vi "custompm.vi"() -> ()   [LabVIEW 2009]
uses:
  <vilib>/Utility/file.llb/Write To Spreadsheet File (DBL).vi
  <vilib>/Analysis/NI_AALBase.lvlib
panel:
  in  "Power Scan File Save Path":path
  in  "Save Scan":bool
  out "XY Graph":cluster{dbl[], dbl[]}(graph)
  out "Wave Cal":dbl
  in  "BWIn":u16(ring) caption="Bandwidth" items=["HIGH", "LOW"]
  in  "Averaging Rate":i32=300 min=1 max=10000 step=1
  in  "Beam\nDiameter (mm)":dbl=1.0 min=1.0 max=9.0 step=0.5
  out "RANG_Val":dbl
  out "RANG_lbl":string
  out "Rng":string
  out "AUTO?":bool
  in  "AUTO":bool
  in  "Range":i16=1 min=1 max=4 step=1
  in  "Zero?":bool
  out "ZeroValue":dbl
  out "Error log":string
  out "Readout string":string
  out "Readout value":dbl format="%^#_9e"
  out "New":bool
  in  "Close Power Meter":bool
  out "PM Visa":refnum<visa-resource-name>
  out "PM Error":errorcluster
  out "Sensor SN":string
  out "Sensor Name":string
  out "Power Meter Active?":bool
  out "IDN String":string
  in  "Use PowerMeter":bool
  out "Turning Turret":bool
  in  "Exit":bool
  in  "Abort\n Scan":bool
  out "Scanning":bool
  out "error out":errorcluster
  out "Status":string
  out "Emulating":bool
  out "Initialized":bool
  in  "Force\nInitialization":bool
  in  "Initialize":bool
  out "Current UniqueID":string
  in  "Mono ID":string(combo)
  in  "Switch \nTurret":bool
  out "Wavelength (nm)":dbl
  out "Grating Index":i32
  in  "Select Grating Blaze":string(combo)
  out "Current Blaze":string caption="Grating Blaze"
  out "Grating Density":dbl
  in  "Step Time (sec)":dbl=1.0 min=0.01 max=10.0 step=0.01
  in  "Wavelength\n   Step Size":dbl=1.0 min=0.1 max=100.0
  in  "Ending\nWavelength":dbl=500.0 min=451.0 max=2501.0
  in  "Starting\nWavelength":dbl=400.0 min=400.0 max=2500.0
  in  "Target\nWavelength":dbl=400.0 min=400.0 max=3000.0
  in  "Increment":dbl=10.0 min=0.1 max=50.0
  out "Incrementing Down":bool
  out "Incrementing Up":bool
  out "Changing Wavelength":bool
  in  "Scan":bool
  in  "Increment Down":bool
  in  "Increment Up":bool
  in  "Change Wavelength":bool
  out "Drive Control Engaged":bool
  in  "Change \nGrating":bool
  in  "Enable\nDrive":bool
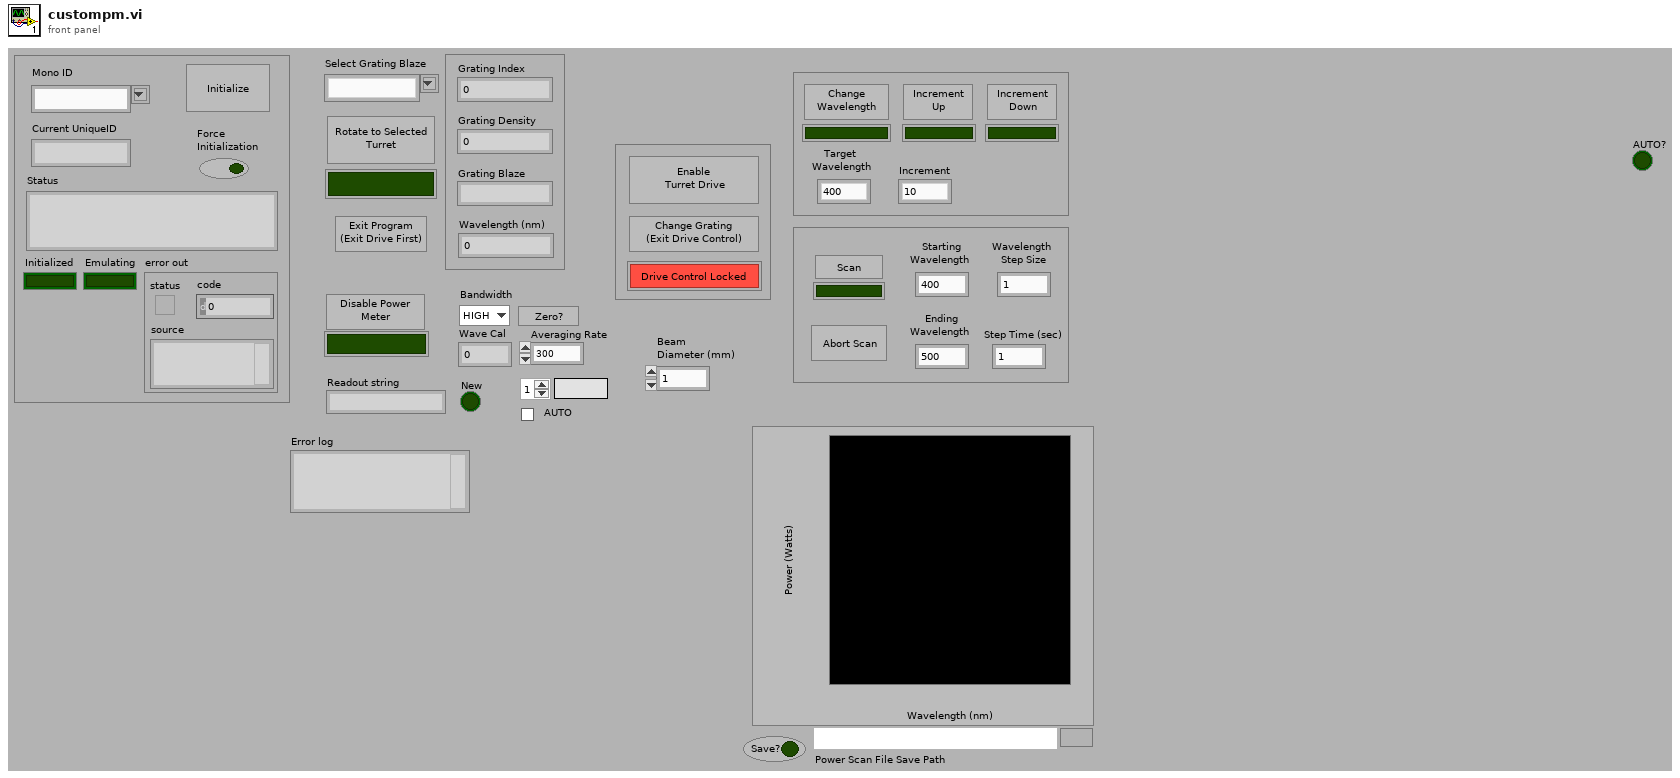
[diagram p1: front panel]
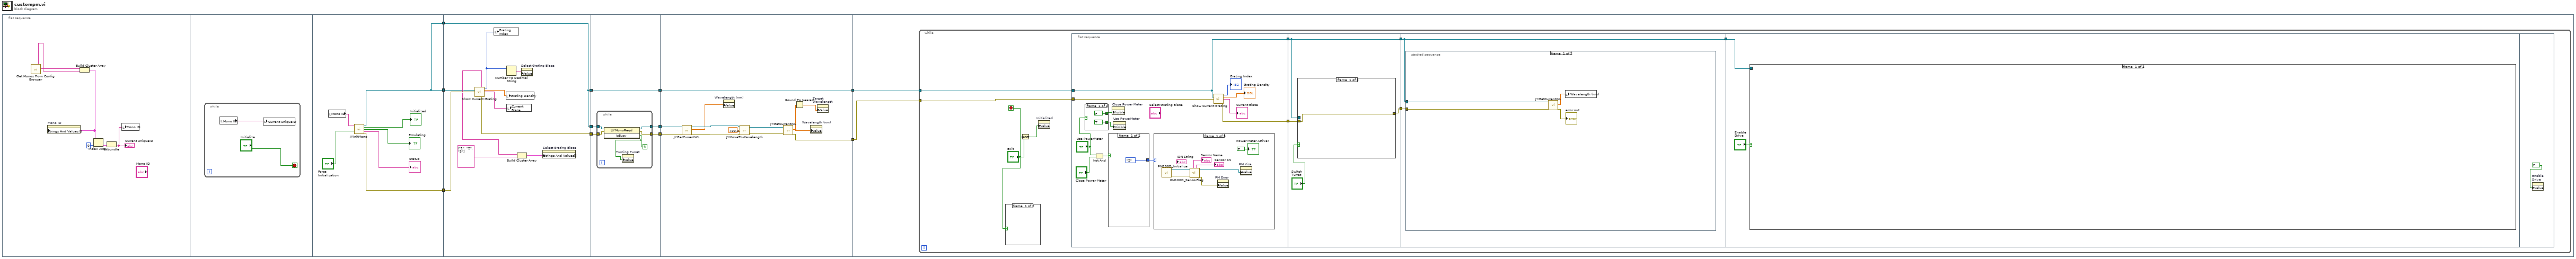
[diagram p0: block diagram]
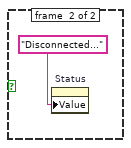
[diagram p2: hidden frame]
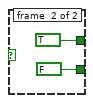
[diagram p3: hidden frame]
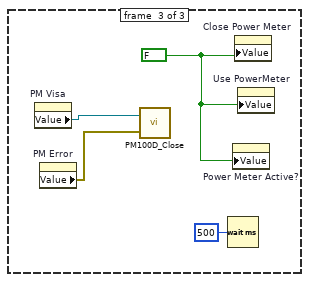
[diagram p5: hidden frame]
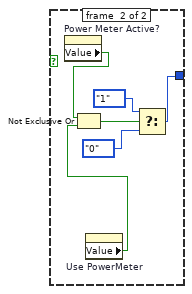
[diagram p6: hidden frame]
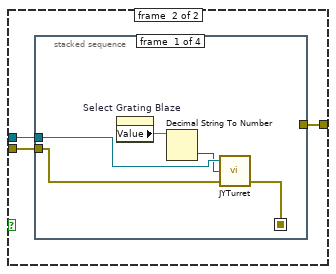
[diagram p7: hidden frame]
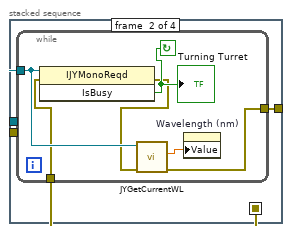
[diagram p8: hidden frame]
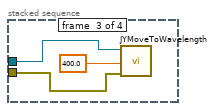
[diagram p9: hidden frame]
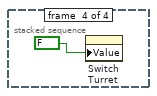
[diagram p10: hidden frame]
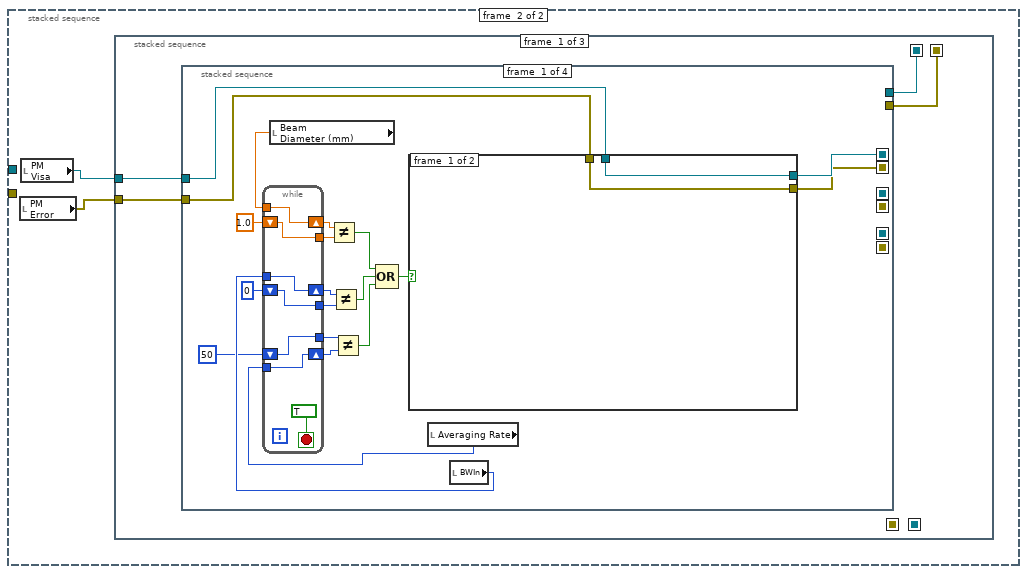
[diagram p11: hidden frame]
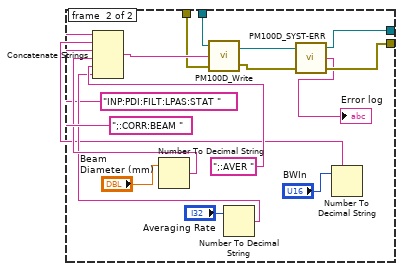
[diagram p12: hidden frame]
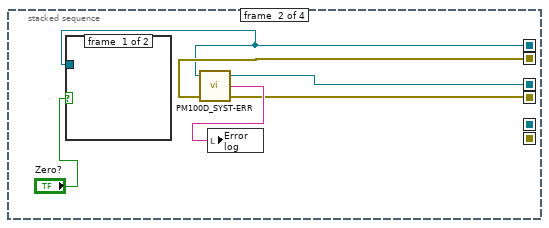
[diagram p13: hidden frame]
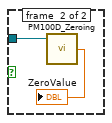
[diagram p14: hidden frame]
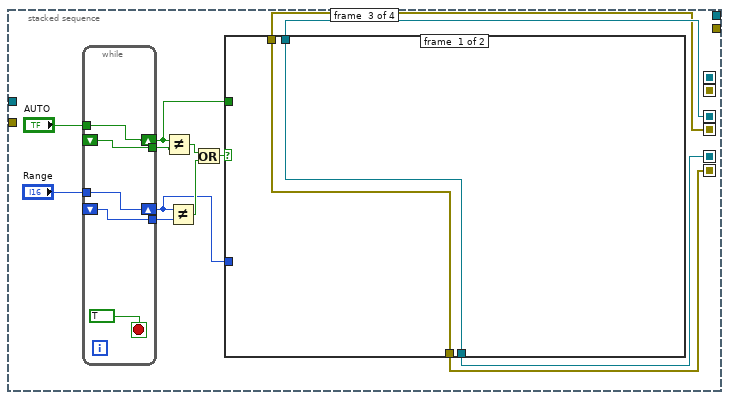
[diagram p15: hidden frame]
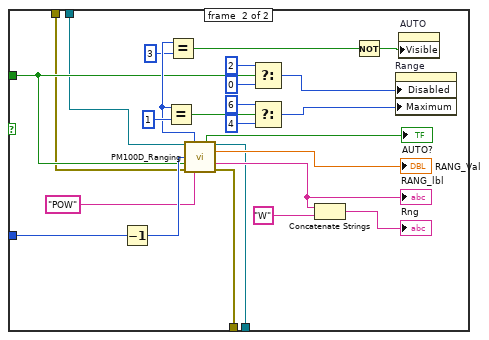
[diagram p16: hidden frame]
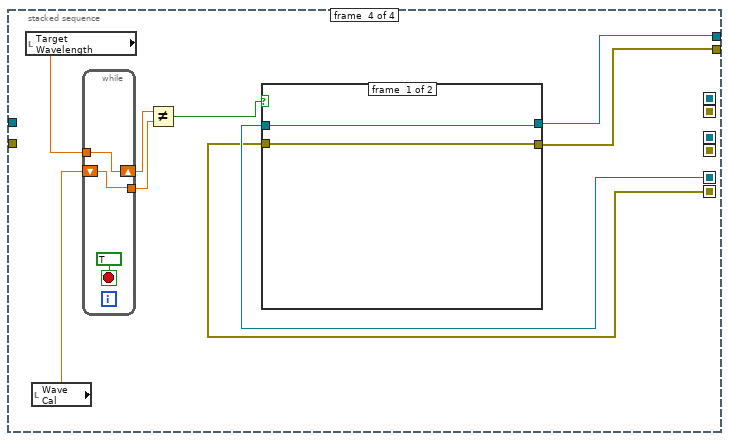
[diagram p17: hidden frame]
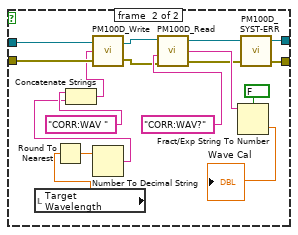
[diagram p18: hidden frame]
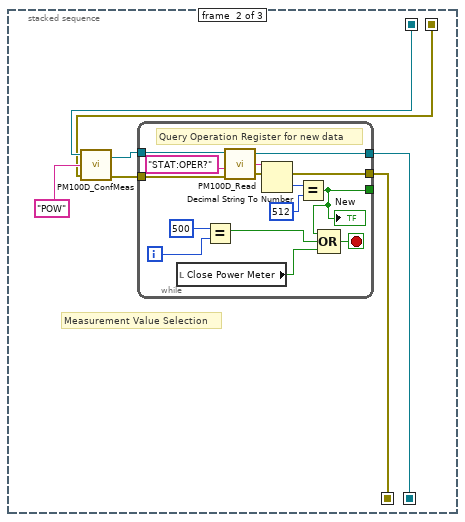
[diagram p19: hidden frame]
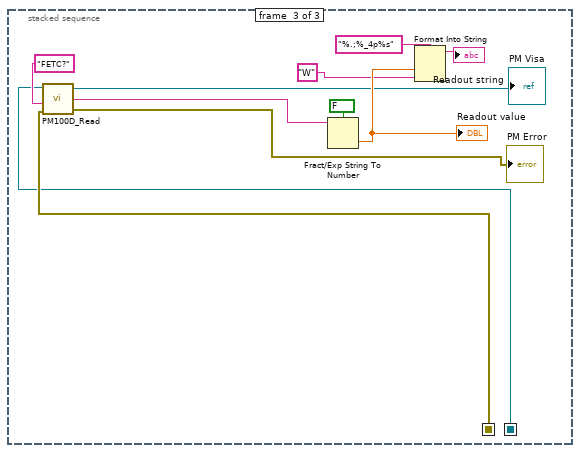
[diagram p20: hidden frame]
diagram:
  n1 = flat-sequence {
    tunnel: [w21] -> w11
    tunnel: [w20] -> w10
    tunnel: [w20] -> w7
    tunnel: w11 -> [w37]
    tunnel: w10 -> [w28]
    tunnel: [w35] -> w4
    tunnel: [w27] -> w6
    tunnel: w7 -> [w27]
    tunnel: [w27] -> w3
    tunnel: w6 -> [w41]
    tunnel: [w39] -> w5
    tunnel: w4 -> [w40]
    tunnel: w3 -> [w42]
    tunnel: [w42] -> w2
    tunnel: [w38] -> w1
    tunnel: w5 -> [w59]
    tunnel: [w57] -> w9
    tunnel: [w56] -> w8
    tunnel: w2 -> [w57]
    tunnel: w1 -> [w58]
    tunnel: w9 -> [w60]
    tunnel: w8 -> [w61]
    frame #0 {
      n2 = call "Get Monos From Config Browser.vi"() -> ("UniqueIDs"=w16:string[], "Mono ID"=w17:string[])  [unwired: 3 in, 1 out]
      n3 = Build Cluster Array(w17, w16) -> (w14:cluster{"String":string, "String":string}[])
      n4 = property on="Mono ID" class="CmbBox"("Strings And Values []"=w14) -> ()  [unwired: 2 in, 2 out]
      n5 = Index Array(array=w14, index=0) -> (element=w15:cluster{"String":string, "String":string})
      n6 = Unbundle(w15) -> ("String"=w12:string)  [unwired: 1 out]
      "Current UniqueID" <- w12
      n7 = local write "Mono ID"(w12) -> ()
    }
    frame #1 {
      n8 = while {
        stop <- "Initialize" stop-if-true
        n9 = local read "Mono ID"() -> (w19:string)
        n10 = local write "Current UniqueID"(w19) -> ()
      }
    }
    frame #2 {
      n11 = local read "Mono ID"() -> (w25:string)
      n12 = call "JYInitMono.vi"("Unique ID"=w25, "Force Init"="Force\nInitialization") -> ("Mono RefNum out"=w20:refnum<k7>, "Initialized"=→"Initialized":bool, "Emulating"=→"Emulating":bool, "Status"=→"Status":string, "error out"=w21:errorcluster)  [unwired: 9 in]
    }
    frame #3 {
      n13 = call "Show Current Grating.vi"("Refnum in"=w28, "error in (no error)"=w37) -> ("Blazes"=w32:string[], "Grating Index"=w31:i32, "Current Grating"=w30:dbl, "Current Blaze"=w29:string, "error out"=w35:errorcluster)  [unwired: 5 in, 4 out]
      n14 = local write "Grating Index"(w31) -> ()
      n15 = local write "Grating Density"(w30) -> ()
      n16 = Number To Decimal String(number=w31) -> (decimal integer string=w34:string)  [unwired: 1 in]
      n17 = local write "Current Blaze"(w29) -> ()
      n18 = Build Cluster Array(w32, string[] ["1", "2", "3"]) -> (w33:cluster{"String":string, string}[])
      n19 = property on="Select Grating Blaze" class="CmbBox"("Value"=w34) -> ()  [unwired: 2 in, 2 out]
      n20 = property on="Select Grating Blaze" class="CmbBox"("Strings And Values[]"=w33) -> ()  [unwired: 2 in, 2 out]
    }
    frame #4 {
      n21 = while {
        tunnel: w41 -> [w47]
        tunnel: w40 -> [w46]
        tunnel: [w45] -> w39
        tunnel: [w44] -> w38
        stop <- w43 continue-if-true
        n22 = invoke class="IJYMonoReqd" method="IsBusy"(reference=w47, error in=w46) -> (reference out=w45:refnum<k7>, error out=w44:errorcluster, "IsBusy"=w43:bool)  [unwired: 1 in]
        n23 = property on="Turning Turret" class="Bool (strict)"("Value"=w43) -> ()  [unwired: 2 in, 2 out]
      }
    }
    frame #5 {
      n24 = call "JYGetCurrentWL.vi"("error in (no error)"=w58, "JYMONOLib.IJYMonoReqd"=w59) -> ("error out"=w53:errorcluster, "Current WL"=w49:dbl, "Mono Refnum Out"=w54:refnum<k7>)  [unwired: 6 in, 1 out]
      n25 = property on="Wavelength (nm)" class="DigNum (strict)"("Value"=w49) -> ()  [unwired: 2 in, 2 out]
      n26 = call "JYMoveToWavelength.vi"("error in (no error)"=w53, "Target WL"=400.0, "RefNum In"=w54) -> ("error out"=w51:errorcluster, "Refnum Out"=w52:refnum<k7>)  [unwired: 1 in, 1 out]
      n27 = call "JYGetCurrentWL.vi"("error in (no error)"=w51, "JYMONOLib.IJYMonoReqd"=w52) -> ("error out"=w56:errorcluster, "Current WL"=w50:dbl)  [unwired: 6 in, 2 out]
      n28 = Round To Nearest(number=w50) -> (nearest integer value=w48:dbl)
      n29 = property on="Wavelength (nm)" class="DigNum (strict)"("Value"=w50) -> ()  [unwired: 2 in, 2 out]
      n30 = property on="Target\nWavelength" class="DigNum (strict)"("Value"=w48) -> ()  [unwired: 2 in, 2 out]
    }
    frame #6 {
      n31 = while {
        tunnel: w60 -> [w70]
        tunnel: w61 -> [w69]
        stop <- "Exit" stop-if-true
        n32 = case shown="True" "Exit" {
          frame #0 {
          }
          frame #1 {
            n33 = property on="Status" class="Str"("Value"="Disconnected...") -> ()  [unwired: 2 in, 2 out]
          }
        }
        n34 = Not(x="Exit") -> (.not. x?=w62:bool)
        n35 = property on="Initialized" class="Bool (strict)"("Value"=w62) -> ()  [unwired: 2 in, 2 out]
        n36 = flat-sequence {
          tunnel: w70 -> [w78]
          tunnel: w69 -> [w80]
          tunnel: [w79] -> w68
          tunnel: [w78] -> w66
          tunnel: w68 -> [w109]
          tunnel: [w107] -> w67
          tunnel: w66 -> [w108]
          tunnel: [w108] -> w65
          tunnel: w67 -> [w133]
          tunnel: w65 -> [w132]
          tunnel: [w132] -> w64
          tunnel: w64 -> [w307]
          frame #0 {
            n37 = case shown="True" "Use PowerMeter" {
              tunnel: [FALSE TRUE] -> w72
              tunnel: [TRUE FALSE] -> w73
              frame #0 {
              }
              frame #1 {
              }
            }
            n38 = Not And(1:"Close Power Meter", 2:"Use PowerMeter") -> (0:w76:bool)
            n39 = case shown="True" w76 {
              tunnel: [enum16{"0", "1", "2"}."2" w102] -> w75
              frame #0 {
              }
              frame #1 {
                n40 = property on="Power Meter Active?" class="Bool (strict)"() -> ("Value"=w100:bool)  [unwired: 2 in, 2 out]
                n41 = property on="Use PowerMeter" class="Bool (strict)"() -> ("Value"=w101:bool)  [unwired: 2 in, 2 out]
                n42 = Not Exclusive Or(1:w101, 2:w100) -> (0:w103:bool)
                n43 = Select(t=enum16{"0", "1", "2"}."1", s=w103, f=enum16{"0", "1", "2"}."0") -> (s? t:f=w102:enum16{"0", "1", "2"})
              }
            }
            n44 = property on="Close Power Meter" class="Bool (strict)"("Visible"=w72) -> ()  [unwired: 2 in, 2 out]
            n45 = property on="Use PowerMeter" class="Bool (strict)"("Visible"=w73) -> ()  [unwired: 2 in, 2 out]
            n46 = case shown="\"2\"" w75 {
              frame #0 {
                n47 = call "PM100D_Initialize.vi"() -> ("error out"=w92:errorcluster, "VISA out"=w93:refnum<visa-resource-name>)  [unwired: 2 in, 2 out]
                n48 = call "PM100D_SensorFlag.vi"("error in (no error)"=w92, "VISA in"=w93) -> ("error out"=w89:errorcluster, "VISA out"=w88:refnum<visa-resource-name>, "sn"=→"Sensor SN":string, "name"=→"Sensor Name":string)  [unwired: 2 in, 4 out]
                n49 = property on="PM Error" class="Clust (strict)"("Value"=w89) -> ()  [unwired: 2 in, 2 out]
                n50 = property on="PM Visa" class="VISAName"("Value"=w88) -> ()  [unwired: 2 in, 2 out]
                "Power Meter Active?" <- TRUE ("Power Meter Active?")
              }
              frame #1 {
              }
              frame #2 {
                w96 = FALSE
                n51 = property on="PM Visa" class="VISAName"() -> ("Value"=w98:refnum<visa-resource-name>)  [unwired: 2 in, 2 out]
                n52 = property on="PM Error" class="Clust (strict)"() -> ("Value"=w97:errorcluster)  [unwired: 2 in, 2 out]
                n53 = call "PM100D_Close.vi"("error in (no error)"=w97, "VISA resource name"=w98) -> ()  [unwired: 2 in]
                n54 = Wait (ms)(milliseconds to wait=u32 500) -> ()  [unwired: 1 out]
                n55 = property on="Power Meter Active?" class="Bool (strict)"("Value"=w96) -> ()  [unwired: 2 in, 2 out]
                n56 = property on="Close Power Meter" class="Bool (strict)"("Value"=w96) -> ()  [unwired: 2 in, 2 out]
                n57 = property on="Use PowerMeter" class="Bool (strict)"("Value"=w96) -> ()  [unwired: 2 in, 2 out]
              }
            }
            n58 = call "Show Current Grating.vi"("Refnum in"=w78, "error in (no error)"=w80) -> ("Grating Index"=→"Grating Index":i32, "Current Grating"=→"Grating Density":dbl, "Current Blaze"=→"Current Blaze":string, "error out"=w79:errorcluster)  [unwired: 5 in, 5 out]
          }
          frame #1 {
            n59 = case shown="True" "Switch \nTurret" {
              tunnel: w109 -> [w110 w113]
              tunnel: w108 -> [_ w112]
              tunnel: [w110 w111] -> w107
              frame #0 {
              }
              frame #1 {
                n60 = stacked-sequence {
                  seq-local: [w116 _ _ _] -> [_ w120 _ _]
                  tunnel: w113 -> [w118 _ w129 _]
                  tunnel: w112 -> [w117 w121 w128 _]
                  tunnel: [_ w119 _ _] -> w111
                  frame #0 {
                    n61 = property on="Select Grating Blaze" class="CmbBox"() -> ("Value"=w115:string)  [unwired: 2 in, 2 out]
                    n62 = Decimal String To Number(string=w115) -> (number=w114:i32)  [unwired: 2 in, 1 out]
                    n63 = call "JYTurret.vi"("error in (no error)"=w118, "Grating Index"=w114, "RefNum In"=w117) -> ("error out"=w116:errorcluster)  [unwired: 2 out]
                  }
                  frame #1 {
                    n64 = while {
                      tunnel: w121 -> [w127]
                      tunnel: w120 -> [w126]
                      tunnel: [w123] -> w119
                      stop <- w125 continue-if-true
                      n65 = invoke class="IJYMonoReqd" method="IsBusy"(reference=w127, error in=w126) -> (error out=w124:errorcluster, "IsBusy"=w125:bool)  [unwired: 1 in, 1 out]
                      "Turning Turret" <- w125
                      n66 = call "JYGetCurrentWL.vi"("error in (no error)"=w124, "JYMONOLib.IJYMonoReqd"=w127) -> ("error out"=w123:errorcluster, "Current WL"=w122:dbl)  [unwired: 6 in, 2 out]
                      n67 = property on="Wavelength (nm)" class="DigNum (strict)"("Value"=w122) -> ()  [unwired: 2 in, 2 out]
                    }
                  }
                  frame #2 {
                    n68 = call "JYMoveToWavelength.vi"("error in (no error)"=w129, "Target WL"=400.0, "RefNum In"=w128) -> ()  [unwired: 1 in, 3 out]
                  }
                  frame #3 {
                    n69 = property on="Switch \nTurret" class="Bool (strict)"("Value"=FALSE ("Switch \nTurret")) -> ()  [unwired: 2 in, 2 out]
                  }
                }
              }
            }
          }
          frame #2 {
            n70 = stacked-sequence {
              tunnel: w133 -> [w137 _]
              tunnel: w132 -> [w136 _]
              frame #0 {
                n71 = call "JYGetCurrentWL.vi"("error in (no error)"=w137, "JYMONOLib.IJYMonoReqd"=w136) -> ("error out"=→"error out":errorcluster, "Current WL"=w134:dbl)  [unwired: 6 in, 2 out]
                n72 = local write "Wavelength (nm)"(w134) -> ()
              }
              frame #1 {
                n73 = local read "PM Error"() -> (w138:errorcluster)
                n74 = local read "PM Visa"() -> (w139:refnum<visa-resource-name>)
                n75 = stacked-sequence {
                  seq-local: [_ w278 _] -> [_ _ w299]
                  seq-local: [_ w277 _] -> [_ _ w298]
                  seq-local: [w141 _ _] -> [_ w275 _]
                  seq-local: [w140 _ _] -> [_ w274 _]
                  tunnel: w139 -> [w143 _ _]
                  tunnel: w138 -> [w142 _ _]
                  frame #0 {
                    n76 = stacked-sequence {
                      seq-local: [w163 _ _ _] -> [_ w193 _ _]
                      seq-local: [w162 _ _ _] -> [_ w194 _ _]
                      seq-local: [_ w191 _ _] -> [_ _ w201 _]
                      seq-local: [_ w190 _ _] -> [_ _ w200 _]
                      seq-local: [_ _ w199 _] -> [_ _ _ w248]
                      seq-local: [_ _ w198 _] -> [_ _ _ w247]
                      tunnel: w143 -> [w161 _ _ _]
                      tunnel: w142 -> [w160 _ _ _]
                      tunnel: [_ _ _ w246] -> w141
                      tunnel: [_ _ _ w245] -> w140
                      frame #0 {
                        n77 = local read "Beam\nDiameter (mm)"() -> (w158:dbl)
                        n78 = local read "Averaging Rate"() -> (w157:i32)
                        n79 = local read "BWIn"() -> (w156:u16)
                        n80 = while {
                          shift-right: [w188] -> w154
                          shift-left: 1.0 ("Beam\nDiameter (mm)") -> [w187]
                          shift-right: [w184] -> w152
                          shift-left: u16 0 ("BWIn") -> [w183]
                          shift-right: [w186] -> w150
                          shift-left: 50 ("Averaging Rate") -> [w185]
                          tunnel: w158 -> [w188]
                          tunnel: [w187] -> w155
                          tunnel: w157 -> [w186]
                          tunnel: [w185] -> w151
                          tunnel: w156 -> [w184]
                          tunnel: [w183] -> w153
                          stop <- TRUE stop-if-true
                        }
                        n81 = Not Equal?(x=w154, y=w155) -> (x != y?=w147:bool)
                        n82 = Not Equal?(x=w152, y=w153) -> (x != y?=w148:bool)
                        n83 = Not Equal?(x=w151, y=w150) -> (x != y?=w149:bool)
                        n84 = Compound Arithmetic op=OR(w147, w148, w149) -> (w159:bool)
                        n85 = case shown="True" w159 {
                          tunnel: [w164 w179] -> w163
                          tunnel: [w165 w178] -> w162
                          tunnel: w161 -> [w164 w167]
                          tunnel: w160 -> [w165 w166]
                          frame #0 {
                          }
                          frame #1 {
                            n86 = Number To Decimal String(number="Beam\nDiameter (mm)") -> (decimal integer string=w175:string)  [unwired: 1 in]
                            n87 = Number To Decimal String(number="Averaging Rate") -> (decimal integer string=w171:string)  [unwired: 1 in]
                            n88 = Number To Decimal String(number="BWIn") -> (decimal integer string=w168:string)  [unwired: 1 in]
                            n89 = Concatenate Strings("INP:PDI:FILT:LPAS:STAT ", w168, ";:CORR:BEAM " ("string"), w175, ";:AVER " ("string"), w171) -> (w182:string)
                            n90 = call "PM100D_Write.vi"("error in (no error)"=w166, "Command"=w182, "VISA in"=w167) -> ("error out"=w180:errorcluster, "VISA out"=w181:refnum<visa-resource-name>)
                            n91 = call "PM100D_SYST-ERR.vi"("error out 2"=w180, "VISA In"=w181) -> ("error out"=w178:errorcluster, "Error"=→"Error log":string, "VISA Out"=w179:refnum<visa-resource-name>)  [unwired: 1 in]
                          }
                        }
                      }
                      frame #1 {
                        n92 = case shown="True" "Zero?" {
                          tunnel: w193 -> [_ w197]
                          frame #0 {
                          }
                          frame #1 {
                            n93 = call "PM100D_Zeroing.vi"("VISA In"=w197) -> ("ZeroValue"=→"ZeroValue":dbl)  [unwired: 4 in]
                          }
                        }
                        n94 = call "PM100D_SYST-ERR.vi"("error out 2"=w194, "VISA In"=w193) -> ("error out"=w190:errorcluster, "Error"=w195:string, "VISA Out"=w191:refnum<visa-resource-name>)  [unwired: 1 in]
                        n95 = local write "Error log"(w195) -> ()
                      }
                      frame #2 {
                        n96 = while {
                          shift-right: [w240] -> w202
                          shift-left: _ -> [w239]
                          shift-right: [w242] -> w203
                          shift-left: _ -> [w241]
                          tunnel: "AUTO" -> [w242]
                          tunnel: [w241] -> w209
                          tunnel: "Range" -> [w240]
                          tunnel: [w239] -> w206
                          stop <- TRUE stop-if-true
                        }
                        n97 = Not Equal?(x=w203, y=w209) -> (x != y?=w208:bool)
                        n98 = Not Equal?(x=w202, y=w206) -> (x != y?=w205:bool)
                        n99 = Or(x=w208, y=w205) -> (x .or. y?=w204:bool)
                        n100 = case shown="True" w204 {
                          tunnel: w203 -> [_ w220]
                          tunnel: w202 -> [_ w219]
                          tunnel: w201 -> [w211 w217]
                          tunnel: w200 -> [w212 w215]
                          tunnel: [w211 w214] -> w199
                          tunnel: [w212 w213] -> w198
                          frame #0 {
                          }
                          frame #1 {
                            n101 = Decrement(x=w219) -> (x-1=w227:i16)
                            n102 = call "PM100D_Ranging.vi"("VISA in"=w217, "Index"=w227, "AUTO"=w220, "error in (no error)"=w215, "Unit"="POW") -> ("SensType"=w226:i32, "AUTO?"=→"AUTO?":bool, "VISA out"=w214:refnum<visa-resource-name>, "RANG_Val"=→"RANG_Val":dbl, "RANG_lbl"=w235:string, "error out"=w213:errorcluster)  [unwired: 3 in, 2 out]
                            "RANG_lbl" <- w235
                            n103 = Equal?(x=w226, y=1) -> (x = y?=w231:bool)
                            n104 = Equal?(x=w226, y=3) -> (x = y?=w221:bool)
                            n105 = Select(t=2, s=w220, f=0) -> (s? t:f=w233:i32)
                            n106 = Select(t=6, s=w231, f=4) -> (s? t:f=w232:i32)
                            n107 = Concatenate Strings(w235, "W") -> (→"Rng":string)
                            n108 = Not(x=w221) -> (.not. x?=w222:bool)
                            n109 = property on="Range" class="DigNum (strict)"("Disabled"=w233, "Maximum"=w232) -> ()  [unwired: 2 in, 2 out]
                            n110 = property on="AUTO" class="Bool (strict)"("Visible"=w222) -> ()  [unwired: 2 in, 2 out]
                          }
                        }
                      }
                      frame #3 {
                        n111 = local read "Target\nWavelength"() -> (w243:dbl)
                        n112 = local read "Wave Cal"() -> (w244:dbl)
                        n113 = while {
                          shift-right: [w272] -> w251
                          shift-left: w244 -> [w271]
                          tunnel: w243 -> [w272]
                          tunnel: [w271] -> w250
                          stop <- TRUE stop-if-true
                        }
                        n114 = Not Equal?(x=w251, y=w250) -> (x != y?=w249:bool)
                        n115 = case shown="True" w249 {
                          tunnel: w248 -> [w253 w268]
                          tunnel: w247 -> [w252 w267]
                          tunnel: [w253 w266] -> w246
                          tunnel: [w252 w265] -> w245
                          frame #0 {
                          }
                          frame #1 {
                            n116 = local read "Target\nWavelength"() -> (w254:dbl)
                            n117 = Round To Nearest(number=w254) -> (nearest integer value=w270:dbl)
                            n118 = Number To Decimal String(number=w270) -> (decimal integer string=w263:string)  [unwired: 1 in]
                            n119 = Concatenate Strings("CORR:WAV " ("string"), w263) -> (w264:string)
                            n120 = call "PM100D_Write.vi"("error in (no error)"=w267, "Command"=w264, "VISA in"=w268) -> ("error out"=w257:errorcluster, "VISA out"=w258:refnum<visa-resource-name>)
                            n121 = call "PM100D_Read.vi"("error in (no error)"=w257, "Command"="CORR:WAV?", "VISA in"=w258) -> ("error out"=w255:errorcluster, "ReadValue"=w259:string, "VISA out"=w256:refnum<visa-resource-name>)  [unwired: 1 in]
                            n122 = Fract/Exp String To Number(use system decimal point (T)=FALSE, string=w259) -> (number=→"Wave Cal":dbl)  [unwired: 2 in, 1 out]
                            n123 = call "PM100D_SYST-ERR.vi"("error out 2"=w255, "VISA In"=w256) -> ("error out"=w265:errorcluster, "VISA Out"=w266:refnum<visa-resource-name>)  [unwired: 1 in, 1 out]
                          }
                        }
                      }
                    }
                  }
                  frame #1 {
                    # "Measurement Value Selection"
                    n124 = call "PM100D_ConfMeas.vi"("error in"=w274, "Conf:"="POW", "VISA In"=w275) -> ("error out"=w279:errorcluster, "dup VISA session"=w280:refnum<visa-resource-name>)
                    n125 = while {
                      tunnel: w280 -> [w290]
                      tunnel: w279 -> [w289]
                      tunnel: [w288] -> w277
                      tunnel: [w287] -> w278
                      tunnel: [w283] -> _
                      i -> [w285]
                      stop <- w286 stop-if-true
                      # "Query Operation Register for new data"
                      n126 = local read "Close Power Meter"() -> (w282:bool)
                      n127 = Equal?(x=500, y=w285) -> (x = y?=w284:bool)
                      n128 = call "PM100D_Read.vi"("error in (no error)"=w289, "Command"="STAT:OPER?", "VISA in"=w290) -> ("error out"=w287:errorcluster, "ReadValue"=w293:string, "VISA out"=w288:refnum<visa-resource-name>)  [unwired: 1 in]
                      n129 = Decimal String To Number(string=w293) -> (number=w292:i32)  [unwired: 2 in, 1 out]
                      n130 = Equal?(x=w292, y=512) -> (x = y?=w283:bool)
                      "New" <- w283
                      n131 = Compound Arithmetic op=OR(w283, w284, w282) -> (w286:bool)
                    }
                  }
                  frame #2 {
                    n132 = call "PM100D_Read.vi"("error in (no error)"=w299, "Command"="FETC?", "VISA in"=w298) -> ("error out"=→"PM Error":errorcluster, "ReadValue"=w304:string, "VISA out"=→"PM Visa":refnum<visa-resource-name>)  [unwired: 1 in]
                    n133 = Fract/Exp String To Number(use system decimal point (T)=FALSE, string=w304) -> (number=w301:dbl)  [unwired: 2 in, 1 out]
                    "Readout value" <- w301
                    n134 = Format Into String(format string="%.;%_4p%s", w301, "W") -> (resulting string=→"Readout string":string)  [unwired: 2 in, 1 out]
                  }
                }
              }
            }
          }
          frame #3 {
            n135 = case shown="True" "Enable\nDrive" {
              selector: "Enable\nDrive" -> [_ w308]
              tunnel: w307 -> [_ w309]
              frame #0 {
              }
              frame #1 {
                n136 = while {
                  tunnel: w308 -> [w311]
                  tunnel: w309 -> [w310]
                  stop <- "Change \nGrating" stop-if-true
                  n137 = Not And(1:"Change \nGrating", 2:w311) -> (0:→"Drive Control Engaged":bool)
                  n138 = stacked-sequence {
                    seq-local: [_ "Change Wavelength" _ _ _ _] -> [_ _ w334 w353 _ _]
                    seq-local: [_ _ "Increment Up" _ _ _] -> [_ _ _ w352 _ _]
                    seq-local: [_ _ _ w347 _ _] -> [_ _ _ _ w368 _]
                    seq-local: [_ _ _ w346 _ _] -> [_ _ _ _ w367 _]
                    seq-local: [w315 _ _ _ _ _] -> [_ w320 _ _ _ _]
                    seq-local: [_ w318 _ _ _ _] -> [_ _ w330 _ _ _]
                    seq-local: [_ _ w328 _ _ _] -> [_ _ _ w345 _ _]
                    seq-local: [_ _ _ w343 _ _] -> [_ _ _ _ w363 _]
                    tunnel: w310 -> [w314 w319 w329 w344 w362 _]
                    frame #0 {
                      n139 = local read "error out"() -> (w317:errorcluster)
                      n140 = call "JYGetCurrentWL.vi"("error in (no error)"=w317, "JYMONOLib.IJYMonoReqd"=w314) -> ("error out"=w315:errorcluster, "Current WL"=→"Wavelength (nm)":dbl)  [unwired: 6 in, 2 out]
                    }
                    frame #1 {
                      n141 = case shown="True" "Change Wavelength" {
                        selector: "Change Wavelength" -> [_ w324]
                        tunnel: w320 -> [w322 w327]
                        tunnel: w319 -> [_ w326]
                        tunnel: [w322 w325] -> w318
                        frame #0 {
                        }
                        frame #1 {
                          n142 = property on="Target\nWavelength" class="DigNum (strict)"() -> ("Value"=w323:dbl)  [unwired: 2 in, 2 out]
                          n143 = call "JYMoveToWavelength.vi"("error in (no error)"=w327, "Target WL"=w323, "RefNum In"=w326) -> ("error out"=w325:errorcluster)  [unwired: 1 in, 2 out]
                          "Changing Wavelength" <- w324
                        }
                      }
                    }
                    frame #2 {
                      n144 = Not(x=w334) -> (.not. x?=w331:bool)
                      n145 = And(x="Increment Up", y=w331) -> (x .and. y?=w333:bool)
                      n146 = case shown="True" w333 {
                        selector: w333 -> [_ w339]
                        tunnel: w330 -> [w335 w342]
                        tunnel: w329 -> [_ w341]
                        tunnel: [w335 w340] -> w328
                        frame #0 {
                        }
                        frame #1 {
                          n147 = property on="Increment" class="DigNum (strict)"() -> ("Value"=w338:dbl)  [unwired: 2 in, 2 out]
                          n148 = property on="Target\nWavelength" class="DigNum (strict)"() -> ("Value"=w337:dbl)  [unwired: 2 in, 2 out]
                          n149 = Add(x=w338, y=w337) -> (x+y=w336:dbl)
                          n150 = call "JYMoveToWavelength.vi"("error in (no error)"=w342, "Target WL"=w336, "RefNum In"=w341) -> ("error out"=w340:errorcluster)  [unwired: 1 in, 2 out]
                          n151 = property on="Target\nWavelength" class="DigNum (strict)"("Value"=w336) -> ()  [unwired: 2 in, 2 out]
                          "Incrementing Up" <- w339
                        }
                      }
                    }
                    frame #3 {
                      n152 = Not(x=w352) -> (.not. x?=w350:bool)
                      n153 = Not(x=w353) -> (.not. x?=w351:bool)
                      n154 = Not(x="Increment Down") -> (.not. x?=w347:bool)
                      n155 = And(x=w350, y=w351) -> (x .and. y?=w346:bool)
                      n156 = And(x="Increment Down", y=w346) -> (x .and. y?=w349:bool)
                      n157 = case shown="True" w349 {
                        selector: w349 -> [_ w357]
                        tunnel: w345 -> [w354 w361]
                        tunnel: w344 -> [_ w360]
                        tunnel: [w354 w359] -> w343
                        frame #0 {
                        }
                        frame #1 {
                          n158 = property on="Target\nWavelength" class="DigNum (strict)"() -> ("Value"=w356:dbl)  [unwired: 2 in, 2 out]
                          n159 = property on="Increment" class="DigNum (strict)"() -> ("Value"=w358:dbl)  [unwired: 2 in, 2 out]
                          n160 = Subtract(x=w356, y=w358) -> (x-y=w355:dbl)
                          n161 = call "JYMoveToWavelength.vi"("error in (no error)"=w361, "Target WL"=w355, "RefNum In"=w360) -> ("error out"=w359:errorcluster)  [unwired: 1 in, 2 out]
                          n162 = property on="Target\nWavelength" class="DigNum (strict)"("Value"=w355) -> ()  [unwired: 2 in, 2 out]
                          "Incrementing Down" <- w357
                        }
                      }
                    }
                    frame #4 {
                      n163 = And(x=w368, y=w367) -> (x .and. y?=w365:bool)
                      n164 = And(x="Scan", y=w365) -> (x .and. y?=w366:bool)
                      n165 = case shown="True" w366 {
                        selector: w366 -> [_ w370]
                        tunnel: w363 -> [_ w372]
                        tunnel: w362 -> [_ w371]
                        frame #0 {
                        }
                        frame #1 {
                          n166 = flat-sequence {
                            tunnel: w372 -> [w387]
                            tunnel: w371 -> [w386]
                            tunnel: w370 -> [w384]
                            tunnel: [w380] -> w369
                            tunnel: w369 -> [w471]
                            frame #0 {
                              w383 = dbl[] []
                              n167 = property on="Starting\nWavelength" class="DigNum (strict)"() -> ("Value"=w378:dbl)  [unwired: 2 in, 2 out]
                              n168 = property on="Ending\nWavelength" class="DigNum (strict)"() -> ("Value"=w379:dbl)  [unwired: 2 in, 2 out]
                              n169 = property on="PM Error" class="Clust (strict)"() -> ("Value"=w375:errorcluster)  [unwired: 2 in, 2 out]
                              n170 = property on="Step Time (sec)" class="DigNum (strict)"() -> ("Value"=w376:dbl)  [unwired: 2 in, 2 out]
                              n171 = property on="Wavelength\n   Step Size" class="DigNum (strict)"() -> ("Value"=w377:dbl)  [unwired: 2 in, 2 out]
                              n172 = Subtract(x=w379, y=w378) -> (x-y=w389:dbl)
                              n173 = Divide(x=w389, y=w377) -> (x/y=w388:dbl)
                              n174 = To Long Integer(number=w388) -> (32bit integer=w385:i32)
                              n175 = property on="PM Visa" class="VISAName"() -> ("Value"=w373:refnum<visa-resource-name>)  [unwired: 2 in, 2 out]
                              n176 = while {
                                tunnel: w378 -> [w404]
                                tunnel: w376 -> [w408]
                                shift-right: [w403] -> _
                                shift-left: w387 -> [w407]
                                tunnel: w386 -> [w406]
                                tunnel: w377 -> [w405]
                                tunnel: w385 -> [w399]
                                shift-right: [w394] -> w374
                                shift-left: w375 -> [w397]
                                tunnel: w373 -> [w396]
                                shift-right: [w392] -> w382
                                shift-left: w383 -> [w395]
                                shift-right: [w391] -> w381
                                shift-left: w383 -> [w393]
                                i -> [w402]
                                stop <- w400 stop-if-true
                                n177 = Less Or Equal?(x=w399, y=w402) -> (x <= y?=w401:bool)
                                n178 = Or(x=w401, y="Abort\n Scan") -> (x .or. y?=w400:bool)
                                n179 = stacked-sequence {
                                seq-local: [w427 _ _] -> [_ w437 _]
                                seq-local: [w414 _ _] -> [_ _ w446]
                                seq-local: [w411 _ _] -> [_ _ w445]
                                tunnel: w408 -> [_ _ w448]
                                tunnel: w407 -> [w434 _ _]
                                tunnel: w406 -> [w433 w438 _]
                                tunnel: w405 -> [w432 _ _]
                                tunnel: w402 -> [w431 _ _]
                                tunnel: w404 -> [w428 _ _]
                                tunnel: [_ w436 _] -> w403
                                tunnel: w397 -> [w423 _ _]
                                tunnel: w396 -> [w422 _ _]
                                tunnel: w395 -> [w413 _ _]
                                tunnel: [w412 _ _] -> w392
                                tunnel: [_ _ w443] -> w394
                                tunnel: w393 -> [_ _ w440]
                                tunnel: [_ _ w439] -> w391
                                frame #0 {
                                n180 = To Double Precision Float(number=w431) -> (double precision float=w430:dbl)
                                n181 = Multiply(x=w430, y=w432) -> (x*y=w429:dbl)
                                n182 = Add(x=w429, y=w428) -> (x+y=w410:dbl)
                                n183 = Build Array (concatenate)(w413, w410) -> (w412:dbl[])
                                n184 = property on="Target\nWavelength" class="DigNum (strict)"("Value"=w410) -> ()  [unwired: 2 in, 2 out]
                                n185 = call "JYMoveToWavelength.vi"("error in (no error)"=w434, "Target WL"=w410, "RefNum In"=w433) -> ("error out"=w427:errorcluster)  [unwired: 1 in, 2 out]
                                n186 = Number To Decimal String(number=w410) -> (decimal integer string=w426:string)  [unwired: 1 in]
                                n187 = Concatenate Strings("CORR:WAV " ("string"), w426) -> (w424:string)
                                n188 = call "PM100D_Write.vi"("error in (no error)"=w423, "Command"=w424, "VISA in"=w422) -> ("error out"=w420:errorcluster, "VISA out"=w419:refnum<visa-resource-name>)
                                n189 = call "PM100D_Read.vi"("error in (no error)"=w420, "Command"="CORR:WAV?", "VISA in"=w419) -> ("error out"=w417:errorcluster, "ReadValue"=w415:string, "VISA out"=w418:refnum<visa-resource-name>)  [unwired: 1 in]
                                n190 = call "PM100D_SYST-ERR.vi"("error out 2"=w417, "VISA In"=w418) -> ("error out"=w411:errorcluster, "VISA Out"=w414:refnum<visa-resource-name>)  [unwired: 1 in, 1 out]
                                n191 = Fract/Exp String To Number(use system decimal point (T)=FALSE, string=w415) -> (number=w409:dbl)  [unwired: 2 in, 1 out]
                                n192 = property on="Wave Cal" class="DigNum (strict)"("Value"=w409) -> ()  [unwired: 2 in, 2 out]
                                }
                                frame #1 {
                                n193 = call "JYGetCurrentWL.vi"("error in (no error)"=w437, "JYMONOLib.IJYMonoReqd"=w438) -> ("error out"=w436:errorcluster, "Current WL"=w435:dbl)  [unwired: 6 in, 2 out]
                                n194 = property on="Wavelength (nm)" class="DigNum (strict)"("Value"=w435) -> ()  [unwired: 2 in, 2 out]
                                }
                                frame #2 {
                                n195 = To Unsigned Long Integer(number=w448) -> (unsigned 32bit integer=w447:u32)
                                n196 = while {
                                tunnel: w447 -> [w464]
                                tunnel: w446 -> [w463]
                                shift-right: [w453] -> w442
                                shift-left: dbl[] [] -> [w455]
                                shift-right: [w452] -> w443
                                shift-left: w445 -> [w462]
                                stop <- w469 stop-if-true
                                n197 = call "Elapsed Time"() -> ("Elapsed Time (s)"=w468:dbl)  [unwired: 12 in, 7 out]
                                n198 = Less?(x=w464, y=w468) -> (x < y?=w467:bool)
                                n199 = Multiply(x=w464, y=1000.0) -> (x*y=w466:dbl)
                                n200 = call "PM100D_Fetch.vi"("VISA In"=w463, "Timeout"=w466, "error in"=w462) -> ("VISA Out"=w460:refnum<visa-resource-name>, "ReadValue"=w458:string, "error out"=w459:errorcluster)  [unwired: 1 out]
                                n201 = property on="Abort\n Scan" class="Bool (strict)"() -> ("Value"=w451:bool)  [unwired: 2 in, 2 out]
                                n202 = call "PM100D_SYST-ERR.vi"("error out 2"=w459, "VISA In"=w460) -> ("error out"=w452:errorcluster, "Error"=w449:string)  [unwired: 1 in, 1 out]
                                n203 = Or(x=w451, y=w467) -> (x .or. y?=w469:bool)
                                n204 = property on="Error log" class="Str"("Value"=w449) -> ()  [unwired: 2 in, 2 out]
                                n205 = Fract/Exp String To Number(use system decimal point (T)=FALSE, string=w458) -> (number=w454:dbl)  [unwired: 2 in, 1 out]
                                n206 = Build Array (concatenate)(w455, w454) -> (w453:dbl[])
                                n207 = Format Into String(format string="%.;%_4p%s", w454, "W") -> (resulting string=w450:string)  [unwired: 2 in, 1 out]
                                n208 = property on="Readout string" class="Str"("Value"=w450) -> ()  [unwired: 2 in, 2 out]
                                }
                                n209 = call <vilib>:"Mean.vi"("X"=w442) -> ("mean"=w441:dbl)  [unwired: 1 out]
                                n210 = Build Array (concatenate)(w440, w441) -> (w439:dbl[])
                                }
                                }
                                n211 = Bundle "Bundle"(w392, w391) -> (→"XY Graph":cluster{dbl[], dbl[]})  [unwired: 1 in]
                              }
                              n212 = property on="PM Error" class="Clust (strict)"("Value"=w374) -> ()  [unwired: 2 in, 2 out]
                              n213 = Build Array(w382, w381) -> (w380:dbl[][])
                              "Scanning" <- w384
                            }
                            frame #1 {
                              n214 = case shown="True" "Save Scan" {
                                tunnel: w471 -> [_ w474]
                                frame #0 {
                                }
                                frame #1 {
                                n215 = call-poly <vilib>:"Write To Spreadsheet File.vi"("2D data"=w474, "file path (dialog if empty)"="Power Scan File Save Path") -> ()  [unwired: 6 in, 1 out]
                                n216 = property on="Save Scan" class="Bool (strict)"("Value"=FALSE ("Save Scan")) -> ()  [unwired: 2 in, 2 out]
                                }
                              }
                            }
                          }
                        }
                      }
                    }
                    frame #5 {
                      w475 = FALSE
                      n217 = property on="Changing Wavelength" class="Bool (strict)"("Value"=w475) -> ()  [unwired: 2 in, 2 out]
                      n218 = property on="Incrementing Up" class="Bool (strict)"("Value"=w475) -> ()  [unwired: 2 in, 2 out]
                      n219 = property on="Scanning" class="Bool (strict)"("Value"=w475) -> ()  [unwired: 2 in, 2 out]
                      n220 = property on="Abort\n Scan" class="Bool (strict)"("Value"=w475) -> ()  [unwired: 2 in, 2 out]
                      n221 = property on="Increment Up" class="Bool (strict)"("Value"=w475) -> ()  [unwired: 2 in, 2 out]
                      n222 = property on="Scan" class="Bool (strict)"("Value"=w475) -> ()  [unwired: 2 in, 2 out]
                      n223 = property on="Incrementing Down" class="Bool (strict)"("Value"=w475) -> ()  [unwired: 2 in, 2 out]
                      n224 = property on="Increment Down" class="Bool (strict)"("Value"=w475) -> ()  [unwired: 2 in, 2 out]
                      n225 = property on="Change Wavelength" class="Bool (strict)"("Value"=w475) -> ()  [unwired: 2 in, 2 out]
                    }
                  }
                }
              }
            }
          }
          frame #4 {
            n226 = property on="Enable\nDrive" class="Bool (strict)"("Value"=FALSE) -> ()  [unwired: 2 in, 2 out]
          }
        }
      }
    }
  }
